vi "Get Document Reference.vi"(8 "error in (no error)":errorcluster, 11 "ooCalc in":refnum<class "ooCalc.lvclass">) -> (0 "error out":errorcluster, 1 "Document":refnum<k24>, 3 "ooCalc out":refnum<class "ooCalc.lvclass">)   [LabVIEW 2009, in "ooCalc.lvclass"]
uses:
  ooCalc.lvclass
  C:/Projets/LAVAG/OpenOfficeRGT/AODL/DLLs/AODL.dll
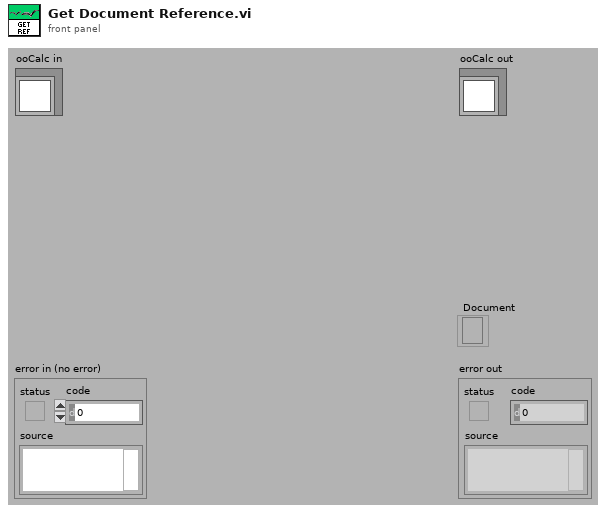
[diagram p1: front panel]
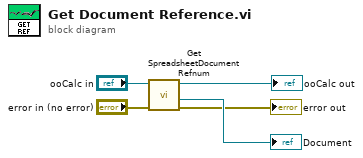
[diagram p0: block diagram]
diagram:
  n1 = call-dynamic "Get SpreadsheetDocument Refnum.vi"("error in (no error)"="error in (no error)", "ooCalc in"="ooCalc in") -> ("error out"=→"error out":errorcluster, "SpreadsheetDocument"=→"Document":refnum<k24>, "ooCalc out"=→"ooCalc out":refnum<class "ooCalc.lvclass">)  [unwired: 7 in]
